vi "ReadAll.vi"(8 "error in (no error)":errorcluster, 11 "connection ID":refnum<k5>) -> (0 "error out":errorcluster, 2 "Read Data":string, 3 "connection ID out":refnum<k5>)   [LabVIEW 2019, in "LifterTCP.lvclass"]
uses:
  LifterTCP.lvclass
panel:
  in  "millisecond multiple":u32=10
  out "Array":string[](array[string])
  out "byte":string
  out "Read end char":bool
  out "status":bool
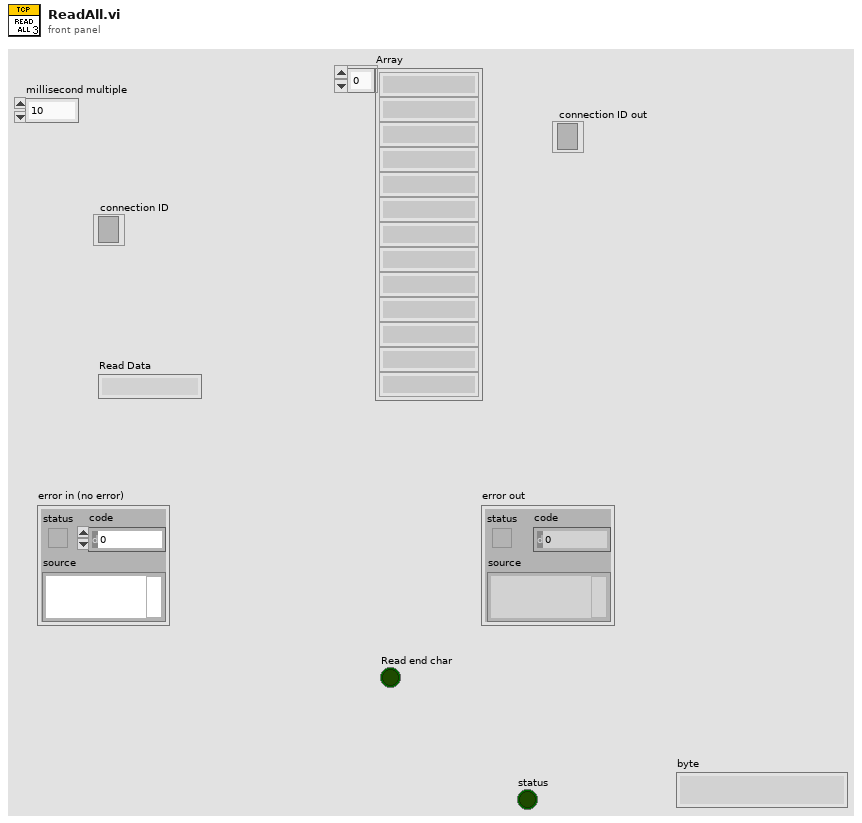
[diagram p1: front panel]
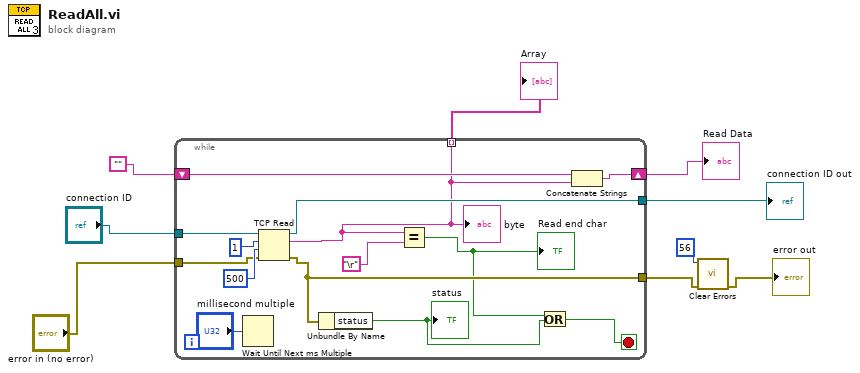
[diagram p0: block diagram]
diagram:
  n1 = while {
    tunnel: [w20] -> w2
    shift-right: [w15] -> w9
    shift-left: "" -> [w16]
    tunnel: [w14] -> w7
    tunnel: "connection ID" -> [w13]
    tunnel: "error in (no error)" -> [w12]
    tunnel: [w11] -> w4 mode=indexing
    stop <- w19 stop-if-true
    n2 = Wait Until Next ms Multiple(millisecond multiple="millisecond multiple") -> ()  [unwired: 1 out]
    n3 = TCP Read(connection ID=w13, bytes to read=1, error in (no error)=w12, 9:500 ("timeout ms (25000)")) -> (connection ID out=w14:refnum<k5>, data out=w11:string, error out=w20:errorcluster)  [unwired: 1 in]
    "byte" <- w11
    n4 = Unbundle By Name(w20) -> ("status"=w18:bool)
    "status" <- w18
    n5 = Equal?(x=w11, y="\r") -> (x = y?=w17:bool)
    "Read end char" <- w17
    n6 = Or(x=w17, y=w18) -> (x .or. y?=w19:bool)
    n7 = Concatenate Strings(w16, w11) -> (w15:string)
  }
  "Read Data" <- w9
  "connection ID out" <- w7
  "Array" <- w4
  n8 = call <vilib>:"Clear Errors.vi"("error in (no error)"=w2, "specific error code to clear (0: all)"=56) -> ("error out"=→"error out":errorcluster)  [unwired: 4 in, 1 out]
